vi "lookuptable_0916.vi"(0 "T_ratio":dbl, 1 "data of 5th order formula\nts,tair,a1-a6 \n(input from the main program)":dbl[](array[numeric]), 3 "step count NM":dbl, 4 "t_shift":dbl=0.000125, 7 "Sample time":i32, 8 "initial":bool, 9 "buffer ratio":dbl, 12 "first or second":bool) -> (6 "output data":bool, 10 "reset step(indicator)":bool, 11 "start to calculate the power":bool, 13 "start to calculate the cost":bool, 14 "Confirm(indicator)":bool, 15 "output cluster 2":T1, 17 "new data of 5th NM":dbl[](array[numeric]), 18 "time180":dbl, 19 "period":dbl)   [LabVIEW 2019]
panel:
  in  "1*8 array":dbl[](array[numeric])
  out "set point":dbl(graph)
  in  "reset step":bool
  in  "confirm that the next 5th data is ok":bool
  out "p_final":dbl
  # "the graph will show up first, \nthen after the confirm boolean \nbecomes true, the new data of \n5th NM will show up"
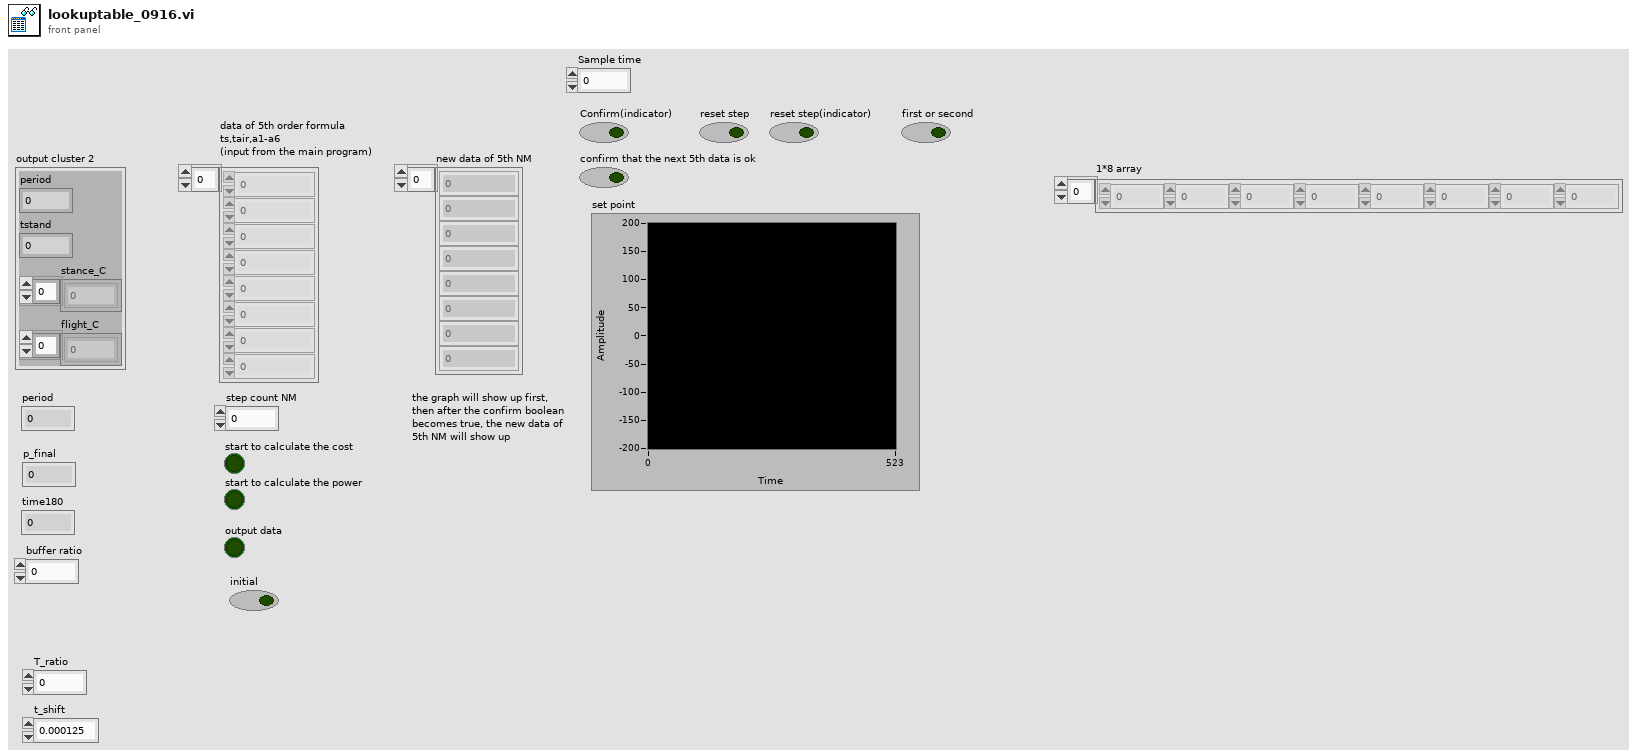
[diagram p1: front panel]
types:
  T1 = cluster{"period":dbl, "tstand":dbl, "stance_C":dbl[], "flight_C":dbl[]}
  T2 = cluster{"Numeric":dbl, "Numeric":dbl, "Numeric":dbl, "Numeric":dbl, "Numeric":dbl, "Numeric":dbl, "Numeric":dbl, "Numeric":dbl}
  T3 = cluster{"number: 0 to 1":dbl, "number: 0 to 1":dbl, "number: 0 to 1":dbl, "number: 0 to 1":dbl, "number: 0 to 1":dbl, "number: 0 to 1":dbl, "number: 0 to 1":dbl, "number: 0 to 1":dbl}
  T4 = cluster{"data of 5th order formula\nts,tair,a1-a6 \n(input from the main program)[0]":dbl, "data of 5th order formula\nts,tair,a1-a6 \n(input from the main program)[1]":dbl, "data of 5th order formula\nts,tair,a1-a6 \n(input from the main program)[2]":dbl, "data of 5th order formula\nts,tair,a1-a6 \n(input from the main program)[3]":dbl, "data of 5th order formula\nts,tair,a1-a6 \n(input from the main program)[4]":dbl, "data of 5th order formula\nts,tair,a1-a6 \n(input from the main program)[5]":dbl, "data of 5th order formula\nts,tair,a1-a6 \n(input from the main program)[6]":dbl, "data of 5th order formula\nts,tair,a1-a6 \n(input from the main program)[7]":dbl, "data of 5th order formula\nts,tair,a1-a6 \n(input from the main program)[8]":dbl}
  T5 = cluster{"pf":dbl, "vf":dbl, dbl, "Numeric":dbl, "Numeric":dbl, "buffer ratio":dbl}
  T6 = cluster{dbl, "Numeric":dbl, dbl[], "flight_C":dbl[]}
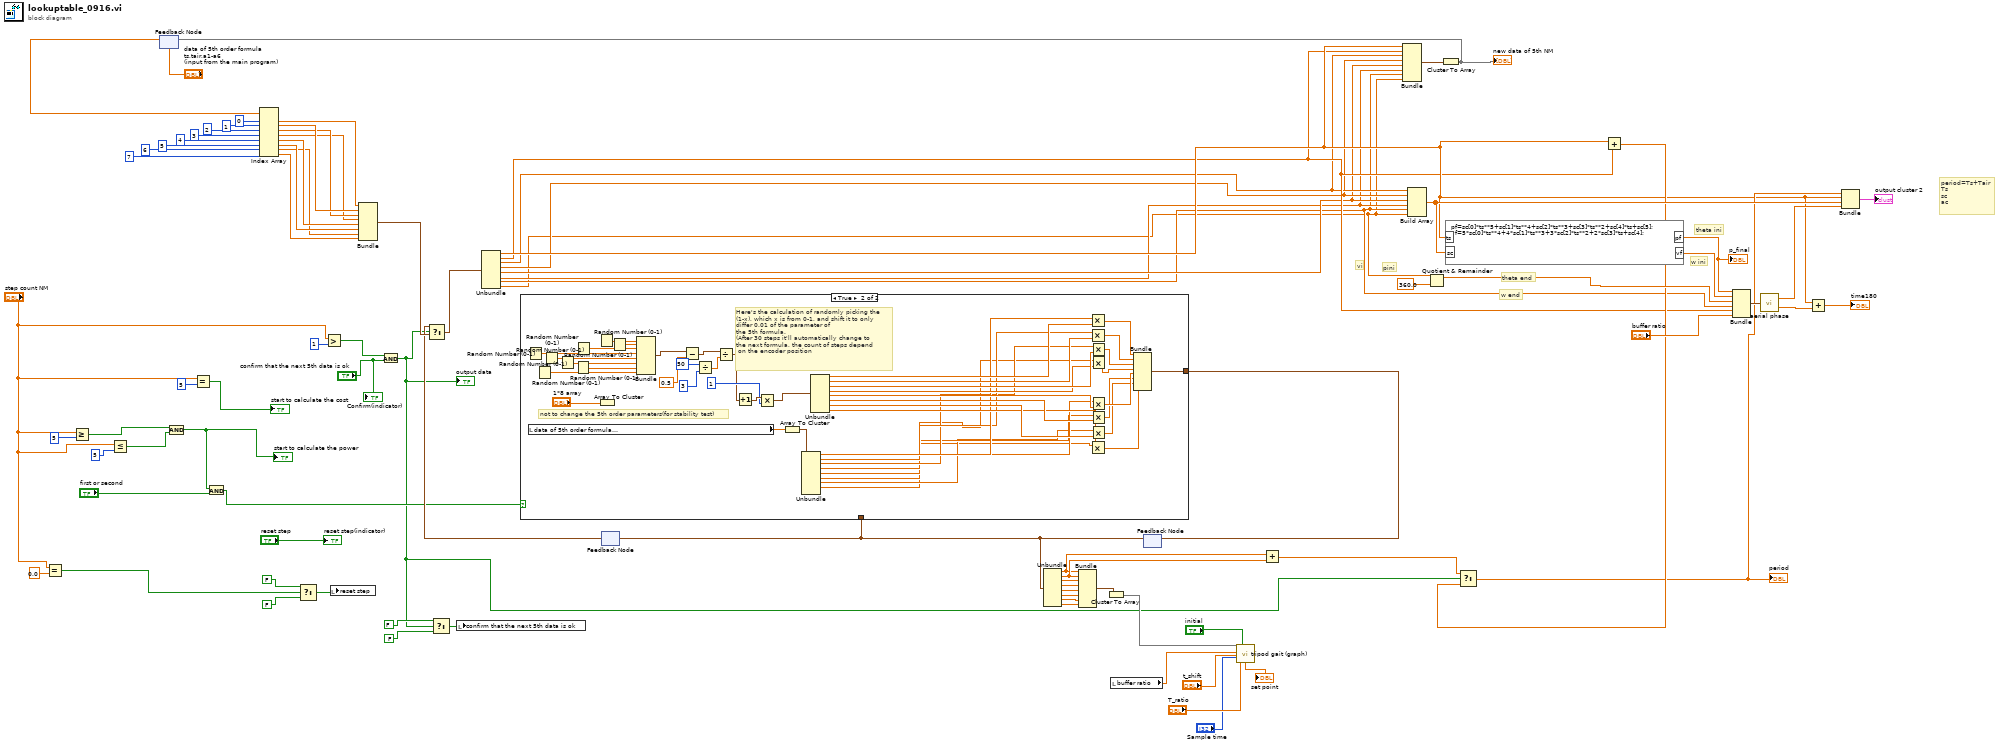
[diagram p0: block diagram]
diagram:
  # "period=Ts+Tair\nTs\nsc\nac"
  # "w ini"
  # "theta ini"
  # "w end"
  # "theta end"
  # "vi"
  # "pini"
  n1 = Equal?(x="step count NM", y=0.0) -> (x = y?=w19:bool)
  n2 = Greater Or Equal?(x="step count NM", y=5) -> (x >= y?=w4:bool)
  n3 = Less Or Equal?(x="step count NM", y=5) -> (x <= y?=w7:bool)
  n4 = feedback #1("data of 5th order formula\nts,tair,a1-a6 \n(input from the main program)") -> (w34:dbl[])
  n5 = And(x=w4, y=w7) -> (x .and. y?=w3:bool)
  "start to calculate the power" <- w3
  n6 = Equal?(x="step count NM", y=5) -> (x = y?=→"start to calculate the cost":bool)
  n7 = And(x=w3, y="first or second") -> (x .and. y?=w18:bool)
  n8 = Index Array "Index Array"(array=w34, index #1=0 ("index"), index #2=1 ("index"), index #3=2 ("index"), index #4=3 ("index"), index #5=4 ("index"), index #6=5 ("index"), index #7=6 ("index"), index #8=7 ("index")) -> (element #1=w66:dbl, element #2=w74:dbl, element #3=w73:dbl, element #4=w72:dbl, element #5=w71:dbl, element #6=w70:dbl, element #7=w69:dbl, element #8=w68:dbl)
  n9 = Select(t=FALSE, s=w19, f=FALSE) -> (s? t:f=w24:bool)
  n10 = Greater?(x="step count NM", y=1) -> (0:w52:bool)
  n11 = local write "reset step"(w24) -> ()
  n12 = Bundle("Numeric"=w66, "Numeric"=w74, "Numeric"=w73, "Numeric"=w72, "Numeric"=w71, "Numeric"=w70, "Numeric"=w69, "Numeric"=w68) -> (w75:T2)  [unwired: 1 in]
  n13 = And(x=w52, y="confirm that the next 5th data is ok") -> (x .and. y?=w11:bool)
  "output data" <- w11
  n14 = Select(t=FALSE, s=w11, f=FALSE) -> (s? t:f=w37:bool)
  n15 = local write "confirm that the next 5th data is ok"(w37) -> ()
  n16 = feedback #2() -> (w67:cluster{dbl, dbl, dbl, dbl, dbl, dbl, dbl, dbl})  [unwired: 1 in]
  n17 = Select(t=w67, s=w11, f=w75) -> (s? t:f=w65:T2)
  n18 = Unbundle(w65) -> ("Numeric"=w51:dbl, "Numeric"=w50:dbl, "Numeric"=w49:dbl, "Numeric"=w48:dbl, "Numeric"=w47:dbl, "Numeric"=w46:dbl, "Numeric"=w45:dbl, "Numeric"=w44:dbl)
  n19 = local read "buffer ratio"() -> (w15:dbl)
  n20 = feedback #3() -> (w32:cluster{dbl, dbl, dbl, dbl, dbl, dbl, dbl, dbl})  [unwired: 1 in]
  n21 = case shown="True" w18 {
    tunnel: [w87 w98] -> w33
    tunnel: w32 -> [w87 _]
    frame False {
    }
    frame True {
      # "not to change the 5th order parameters(for stability test)"
      # "Here's the calculation of randomly picking the \n(1-x), which x is from 0-1, and shift it to only \ndiffer 0.01 of the parameter of \nthe 5th formula.\n(After 30 steps it'll automatically change to \nthe next formula, the count of steps depend\n on the encoder position"
      n22 = Random Number (0-1)() -> (number: 0 to 1=w132:dbl)
      n23 = local read "data of 5th order formula\nts,tair,a1-a6 \n(input from the main program)"() -> (w122:dbl[])
      n24 = Random Number (0-1)() -> (number: 0 to 1=w128:dbl)
      n25 = Random Number (0-1)() -> (number: 0 to 1=w131:dbl)
      n26 = Random Number (0-1)() -> (number: 0 to 1=w130:dbl)
      n27 = Random Number (0-1)() -> (number: 0 to 1=w129:dbl)
      n28 = Random Number (0-1)() -> (number: 0 to 1=w133:dbl)
      n29 = Random Number (0-1)() -> (number: 0 to 1=w127:dbl)
      n30 = Array To Cluster(array="1*8 array") -> ()  [unwired: 1 out]
      n31 = Random Number (0-1)() -> (number: 0 to 1=w126:dbl)
      n32 = Bundle("number: 0 to 1"=w127, "number: 0 to 1"=w126, "number: 0 to 1"=w133, "number: 0 to 1"=w132, "number: 0 to 1"=w131, "number: 0 to 1"=w130, "number: 0 to 1"=w129, "number: 0 to 1"=w128) -> (w123:T3)  [unwired: 1 in]
      n33 = Subtract(x=w123, y=0.5) -> (x-y=w124:T3)
      n34 = Divide(x=50, y=3) -> (x/y=w92:dbl)
      n35 = Divide(x=w124, y=w92) -> (x/y=w88:T3)
      n36 = Increment(x=w88) -> (x+1=w95:T3)
      n37 = Multiply(x=w95, y=1) -> (x*y=w93:T3)
      n38 = Array To Cluster(array=w122) -> (cluster=w105:T4)
      n39 = Unbundle(w105) -> ("data of 5th order formula\nts,tair,a1-a6 \n(input from the main program)[0]"=w113:dbl, "data of 5th order formula\nts,tair,a1-a6 \n(input from the main program)[1]"=w112:dbl, "data of 5th order formula\nts,tair,a1-a6 \n(input from the main program)[2]"=w111:dbl, "data of 5th order formula\nts,tair,a1-a6 \n(input from the main program)[3]"=w110:dbl, "data of 5th order formula\nts,tair,a1-a6 \n(input from the main program)[4]"=w109:dbl, "data of 5th order formula\nts,tair,a1-a6 \n(input from the main program)[5]"=w108:dbl, "data of 5th order formula\nts,tair,a1-a6 \n(input from the main program)[6]"=w107:dbl, "data of 5th order formula\nts,tair,a1-a6 \n(input from the main program)[7]"=w106:dbl)  [unwired: 1 out]
      n40 = Unbundle(w93) -> ("number: 0 to 1"=w121:dbl, "number: 0 to 1"=w120:dbl, "number: 0 to 1"=w119:dbl, "number: 0 to 1"=w118:dbl, "number: 0 to 1"=w117:dbl, "number: 0 to 1"=w116:dbl, "number: 0 to 1"=w115:dbl, "number: 0 to 1"=w114:dbl)
      n41 = Multiply(x=w113, y=w121) -> (x*y=w97:dbl)
      n42 = Multiply(x=w112, y=w120) -> (x*y=w96:dbl)
      n43 = Multiply(x=w106, y=w114) -> (x*y=w99:dbl)
      n44 = Multiply(x=w111, y=w119) -> (x*y=w104:dbl)
      n45 = Multiply(x=w110, y=w118) -> (x*y=w103:dbl)
      n46 = Multiply(x=w109, y=w117) -> (x*y=w102:dbl)
      n47 = Multiply(x=w108, y=w116) -> (x*y=w101:dbl)
      n48 = Multiply(x=w107, y=w115) -> (x*y=w100:dbl)
      n49 = Bundle(w97, w96, w104, w103, w102, w101, w100, w99) -> (w98:cluster{dbl, dbl, dbl, dbl, dbl, dbl, dbl, dbl})  [unwired: 1 in]
    }
  }
  n50 = feedback-in #2(w32) -> ()
  n51 = Unbundle(w32) -> (w1:dbl, w2:dbl, w31:dbl, w30:dbl, w29:dbl, w28:dbl, w27:dbl, w26:dbl)
  n52 = Bundle(w1, w2, w31, w30, w29, w28, w27, w26) -> (w41:cluster{dbl, dbl, dbl, dbl, dbl, dbl, dbl, dbl})  [unwired: 1 in]
  n53 = Cluster To Array(cluster=w41) -> (array=w16:dbl[])
  n54 = feedback-in #3(w33) -> ()
  n55 = call "tripod gait (graph).vi"("data of 5th order formula\nts,tair,a1-a6"=w16, "buffer ratio"=w15, "t_shift"="t_shift", "sample time"="Sample time", "T_ratio"="T_ratio", "initial"="initial") -> ("set point"=→"set point":dbl)  [unwired: 18 in, 3 out]
  n56 = Add(x=w1, y=w2) -> (x+y=w56:dbl)
  n57 = Bundle("Numeric"=w51, "Numeric"=w50, "Numeric"=w49, "Numeric"=w48, "Numeric"=w47, "Numeric"=w46, "Numeric"=w45, "Numeric"=w44) -> (w43:T2)  [unwired: 1 in]
  n58 = Build Array(w49, w48, w47, w46, w45, w44) -> (w80:dbl[])
  n59 = Quotient & Remainder(x=w44, y=360.0) -> (x-y*floor(x/y)=w76:dbl)  [unwired: 1 out]
  n60 = Cluster To Array(cluster=w43) -> (array=w42:dbl[])
  "new data of 5th NM" <- w42
  n61 = feedback-in #1(w42) -> ()
  n62 = formula code="pf=sc[0]*ts**5+sc[1]*ts**4+sc[2]*ts**3+sc[3]*ts**2+sc[4]*ts+sc[5];\nvf=5*sc[0]*ts**4+4*sc[1]*ts**3+3*sc[2]*ts**2+2*sc[3]*ts+sc[4];"("sc"=w80, "ts"=w51) -> ("pf"=w83:dbl, "vf"=w78:dbl)
  "p_final" <- w83
  n63 = Add(x=w51, y=w50) -> (x+y=w55:dbl)
  n64 = Select(t=w56, s=w11, f=w55) -> (s? t:f=w54:dbl)
  "period" <- w54
  n65 = Bundle("pf"=w83, "vf"=w78, w76, "Numeric"=w45, "Numeric"=w50, "buffer ratio"="buffer ratio") -> (w82:T5)  [unwired: 1 out]
  n66 = call "aerial phase.vi"("aerial condition"=w82) -> ("time180"=w81:dbl, "flight_C"=w79:dbl[])  [unwired: 2 in]
  n67 = Add(x=w51, y=w81) -> (x+y=→"time180":dbl)
  n68 = Bundle(w54, "Numeric"=w51, w80, "flight_C"=w79) -> (→"output cluster 2":T6)  [unwired: 1 in]
  "Confirm(indicator)" <- "confirm that the next 5th data is ok"
  "reset step(indicator)" <- "reset step"
